vi "Stop All Child Node.vi"(8 "error in (no error)":errorcluster, 11 "Root Actor in":refnum<class "Root Actor.lvclass">) -> (0 "error out":errorcluster, 3 "Root Actor out":refnum<class "Root Actor.lvclass">)   [LabVIEW 2024, in "Root Actor.lvclass"]
uses:
  Root Actor.lvclass
  Message/Message.lvclass
  Message/Type Def/CMD Type.ctl
  Message/Type Def/General CMD.ctl
  Root Actor.lvclass/Root Actor.ctl
  Message/Message.lvclass/Message.ctl
  Message/Public Data/Write CMD Type.vi
  Message/Public Data/Write General CMD.vi
  Messenger/Messenger/Messenger.lvclass
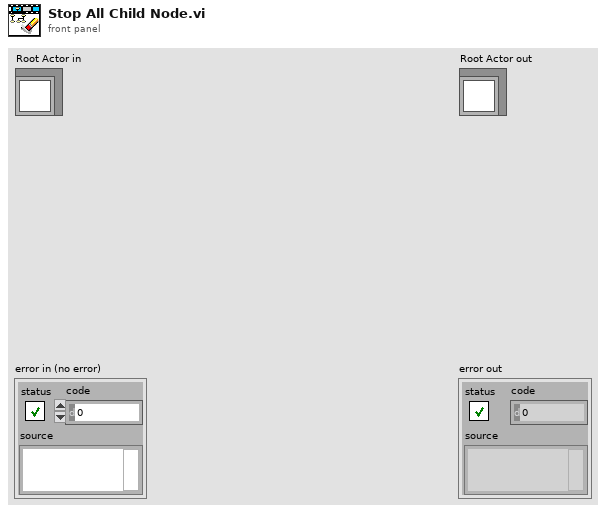
[diagram p1: front panel]
types:
  T1 = typedef "General CMD.ctl" = enum16{"None", "Stop", "Abort", "Running Task", "Running Batch Tasks", "Task Self Running", "Emergency Stop", "Subscribe", "UnSubscribe", "Pause", "Receive Parameters", "Active"}
  T2 = typedef "CMD Type.ctl" = enum16{"None", "General CMD", "1st CMD", "2nd CMD", "3rd CMD", "4th CMD", "5th CMD", "6th CMD", "7th CMD"}
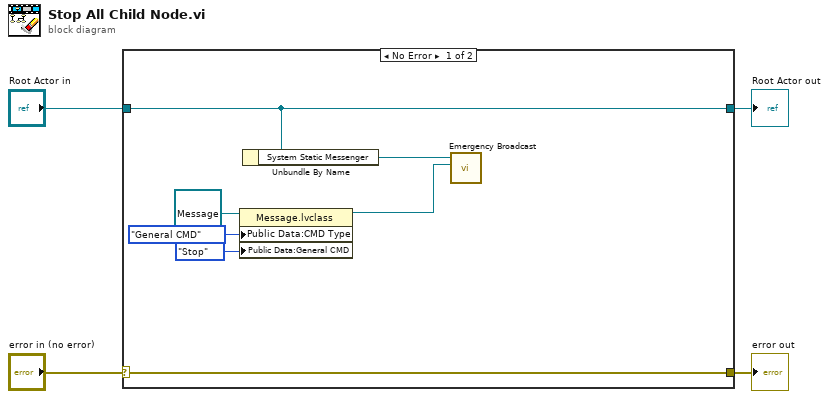
[diagram p0: block diagram]
diagram:
  n1 = case shown="No Error" "error in (no error)" {
    selector: "error in (no error)" -> [w11 w13]
    tunnel: [w11 w13] -> w3
    tunnel: [w10 w12] -> w1
    tunnel: "Root Actor in" -> [w10 w12]
    frame No Error {
      n2 = property class="Message.lvclass"(reference=refnum<class "Message.lvclass"> refnum ("Message In"), "Public Data:CMD Type"=CMD_Type."General CMD" ("CMD Type"), "Public Data:General CMD"=General_CMD."Stop" ("General CMD")) -> (reference out=w5:refnum<class "Message.lvclass">)  [unwired: 1 in, 1 out]
      n3 = Unbundle By Name(w10) -> ("System Static Messenger"=w9:refnum<class "Messenger.lvclass">)
      n4 = call-dynamic "Emergency Broadcast.vi"("Message In"=w5, "Messenger in"=w9) -> ()  [unwired: 8 in, 2 out]
    }
    frame Error {
    }
  }
  "error out" <- w3
  "Root Actor out" <- w1
